vi "connectionStatusString.vi"(7 "connected? [T]":bool=TRUE, 9 "device type":T1 items=["any"=0, "AB1002"=1002, "AB1004"=1004, "AB1502"=1502, "AB1504"=1504, "AB2002"=2002, "AB2004"=2004, "AB2502"=2502, "AB2504"=2504], 10 "Abacus VISA":refnum<visa-resource-name>) -> (1 "String":string)   [LabVIEW 2015]
doc: "Returns a string with the device type, port and its connection status."
uses:
  <instrlib>/Tausand AB1000/Public/Controls/deviceTypeRing.ctl
  <instrlib>/Tausand AB1000/Tausand AB1000.lvlib
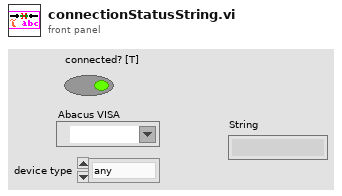
[diagram p1: front panel]
types:
  T1 = typedef "Tausand AB1000.lvlib/deviceTypeRing.ctl" = u16
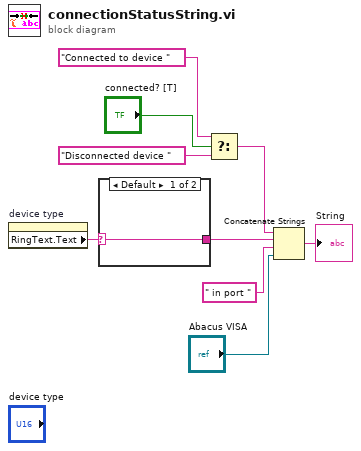
[diagram p0: block diagram]
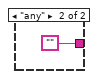
[diagram p2: hidden frame]
diagram:
  n1 = property on="device type" class="Ring (strict)"() -> ("RingText.Text"=w2:string)  [unwired: 2 in, 2 out]
  n2 = case shown="Default" w2 {
    selector: w2 -> [w10 _]
    tunnel: [w10 ""] -> w1
    frame Default {
    }
    frame "any" {
    }
  }
  n3 = Select(t="Connected to device " ("message (overides settings)"), s="connected? [T]", f="Disconnected device " ("message (overides settings)")) -> (s? t:f=w4:string)
  n4 = Concatenate Strings(w4, w1, " in port " ("message (overides settings)"), "Abacus VISA") -> (→"String":string)
